vi "call_alg.vi"(7 "Algorithm name":string, 8 "error in":errorcluster) -> (0 "error out":errorcluster)   [LabVIEW 2013]
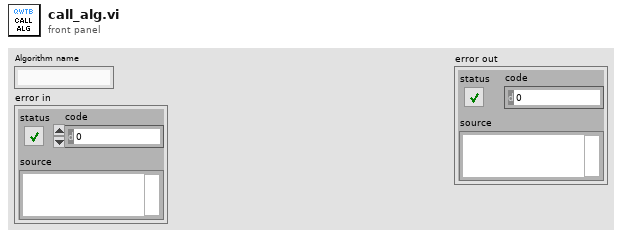
[diagram p1: front panel]
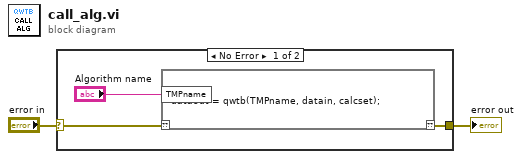
[diagram p0: block diagram]
diagram:
  n1 = case shown="No Error" "error in" {
    selector: "error in" -> [w4 w6]
    tunnel: [w5 w6] -> w2
    frame No Error {
      n2 = script code="dataout = qwtb(TMPname, datain, calcset);"("??"=w4, "TMPname"="Algorithm name") -> ("??"=w5:errorcluster)
    }
    frame Error {
    }
  }
  "error out" <- w2
